vi "instr_initialize.vi"(8 "error in (no error)":errorcluster) -> (0 "error out":errorcluster, 3 "Instrument out":refnum<class "Instrument.lvclass">)   [LabVIEW 2019, in "Instrument.lvclass"]
uses:
  Instrument.lvclass
  Instrument.lvclass/Instrument.ctl
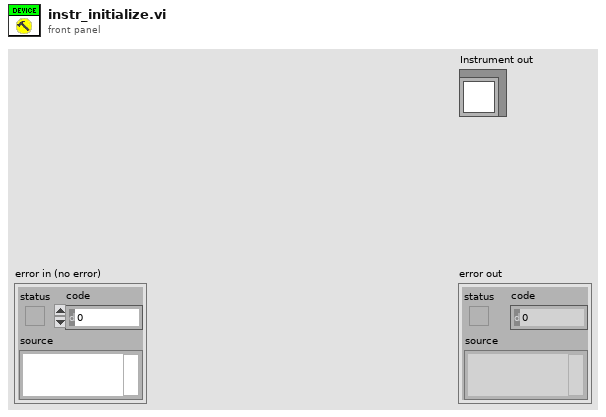
[diagram p1: front panel]
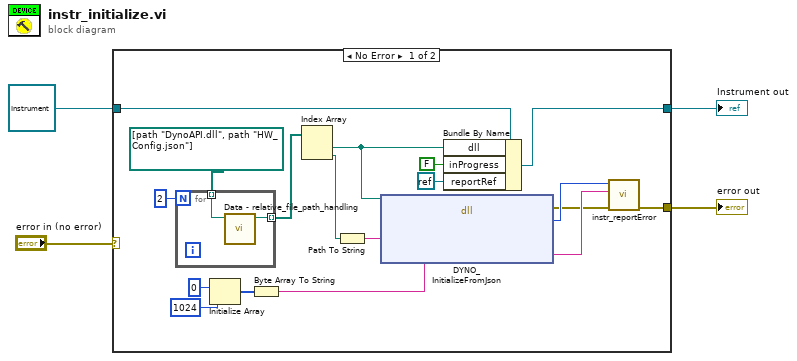
[diagram p0: block diagram]
diagram:
  n1 = case shown="No Error" "error in (no error)" {
    selector: "error in (no error)" -> [_ w26]
    tunnel: [w15 w26] -> w3
    tunnel: [w12 w25] -> w1
    tunnel: refnum<class "Instrument.lvclass"> refnum ("Instrument in") -> [w14 w25]
    frame No Error {
      n2 = for {
        N: 2 -> [_]
        tunnel: [w24] -> w21 mode=indexing
        tunnel: path[] [path "DynoAPI.dll", path "HW_Config.json"] -> [w23] mode=indexing
        n3 = call "Data - relative_file_path_handling.vi"("path in"=w23) -> ("path out"=w24:path)  [unwired: 9 in, 1 out]
      }
      n4 = Initialize Array(u8 0 ("element"), 1024 ("dimension size")) -> (w8:u8[])
      n5 = Byte Array To String(unsigned byte array=w8) -> (string=w9:string)
      n6 = Index Array(array=w21) -> (element #1=w13:path, element #2=w19:path)  [unwired: 2 in]
      n7 = Path To String(path=w19) -> (string=w20:string)
      n8 = dll-call lib="C:/Dev/22KW-Dyno/software/data/DynoAPI.dll" fn="DYNO_InitializeFromJson"(path in=w13, "jsonPath"=w20, "errorMsg"=w9) -> (error out=w16:errorcluster, "return type"=w18:i32, "errorMsg"=w17:string)  [unwired: 3 in, 1 out]
      n9 = Bundle By Name(cluster=w14, "dll"=w13, "inProgress"=FALSE, "reportRef"=refnum<k0> refnum) -> (w12:refnum<class "Instrument.lvclass">)
      n10 = call "instr_reportError.vi"("error in (no error)"=w16, "errorMsg"=w17, "return type"=w18) -> ("error out"=w15:errorcluster)  [unwired: 8 in]
    }
    frame Error {
    }
  }
  "error out" <- w3
  "Instrument out" <- w1
